vi "Scan Test.vi"() -> ()   [LabVIEW 2013]
uses:
  Program Files/National Instruments/LabVIEW 2013/examples/Instrument IO/Serial/support/Serial - Settings.ctl
  <vilib>/Instr/_visa.llb/VISA Configure Serial Port (Instr).vi
panel:
  out "機種代號":string
  out "機種名":string
  in  "stop":bool
  in  "Serial Settings":T1={"baud rate"=9600, "data bits"=8, "parity"=enum."None", "stop bits"=10, "flow control"=0} {"flow control" items=["None"=0, "XON/XOFF"=1, "RTS/CTS"=2, "DTR/DSR"=4]; "stop bits" items=["1.0"=10, "1.5"=15, "2.0"=20]; "data bits" min=5 max=8 step=1; "baud rate" items=["75"=75, "110"=110, "134"=134, "150"=150, "300"=300, "600"=600, "1200"=1200, "1800"=1800, "2400"=2400, "4800"=4800, "7200"=7200, "9600"=9600, "14400"=14400, "19200"=19200, "28800"=28800, "38400"=38400, "56000"=56000, "57600"=57600, "115200"=115200, "128000"=128000, "230400"=230400]}
  out "bytes read":u32
  out "Response":string
  in  "delay before read (ms)":u32=500
  in  "VISA resource name":refnum<visa-resource-name>="COM1"
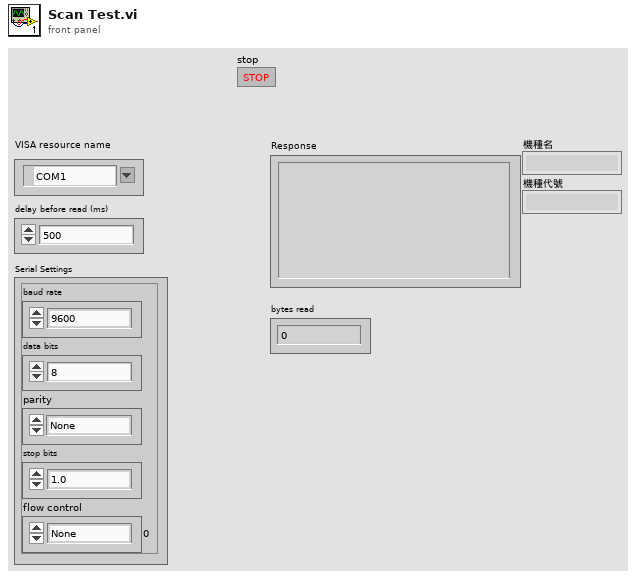
[diagram p1: front panel]
types:
  T1 = typedef "Serial - Settings.ctl" = cluster{"baud rate":u32, "data bits":u16, "parity":enum16{"None", "Odd", "Even", "Mark", "Space"}, "stop bits":u16, "flow control":u16}
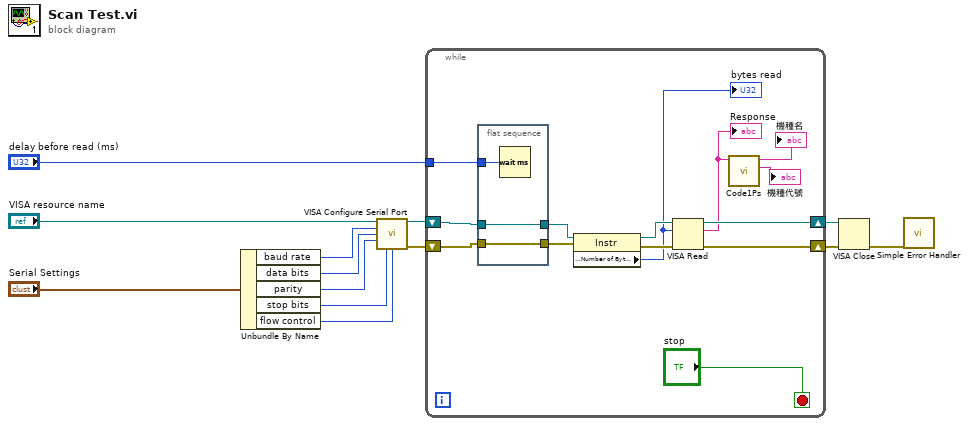
[diagram p0: block diagram]
diagram:
  n1 = Unbundle By Name("Serial Settings") -> ("baud rate"=w7:u32, "data bits"=w6:u16, "parity"=w5:enum16{"None", "Odd", "Even", "Mark", "Space"}, "stop bits"=w4:u16, "flow control"=w3:u16)
  n2 = call-poly "VISA Configure Serial Port"("VISA resource name"="VISA resource name", "baud rate (9600)"=w7, "data bits (8)"=w6, "parity (0:none)"=w5, "stop bits (10: 1 bit)"=w4, "flow control (0:none)"=w3) -> ("VISA resource name out"=w2:refnum<visa-resource-name>, "error out"=w1:errorcluster)  [unwired: 3 in, 5 out]
  n3 = while {
    tunnel: "delay before read (ms)" -> [w25]
    shift-right: [w27] -> w12
    shift-left: w1 -> [w18]
    shift-right: [w26] -> w11
    shift-left: w2 -> [w20]
    stop <- "stop" stop-if-true
    n4 = flat-sequence {
      tunnel: w25 -> [w30]
      tunnel: w20 -> [w29]
      tunnel: [w29] -> w19
      tunnel: w18 -> [w28]
      tunnel: [w28] -> w17
      frame #0 {
        n5 = Wait (ms)(milliseconds to wait=w30) -> ()  [unwired: 1 out]
      }
    }
    n6 = property class="Instr"(reference=w19, error in=w17) -> (reference out=w24:refnum<visa-resource-name>, error out=w23:errorcluster, "Serial Settings:Number of Bytes at Serial Port"=w22:u32)
    "bytes read" <- w22
    n7 = VISA Read(VISA resource name=w24, byte count=w22, error in (no error)=w23) -> (VISA resource name out=w26:refnum<visa-resource-name>, read buffer=w16:string, error out=w27:errorcluster)  [unwired: 1 out]
    "Response" <- w16
    n8 = call "Code1Ps.vi"("Code1 In"=w16) -> ("機種代號"=→"機種代號":string, "機種名"=→"機種名":string)  [unwired: 9 in]
  }
  n9 = VISA Close(VISA resource name=w11, error in (no error)=w12) -> (error out=w10:errorcluster)
  n10 = call <vilib>:"Simple Error Handler.vi"("error in (no error)"=w10) -> ()  [unwired: 1 in, 8 out]
